vi "Calculate_Sensitivity.vi"(8 "Min Sensitivity":dbl, 9 "Current RPM":dbl, 10 "Max Sensitivity":dbl, 11 "Max RPM":dbl) -> (3 "Sensitivity":dbl)   [LabVIEW 2017]
panel:
  in  "stop":bool=TRUE
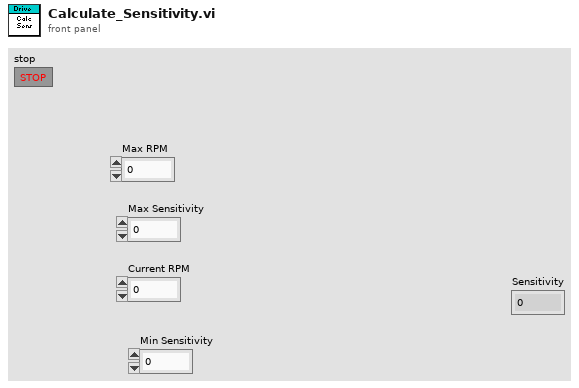
[diagram p1: front panel]
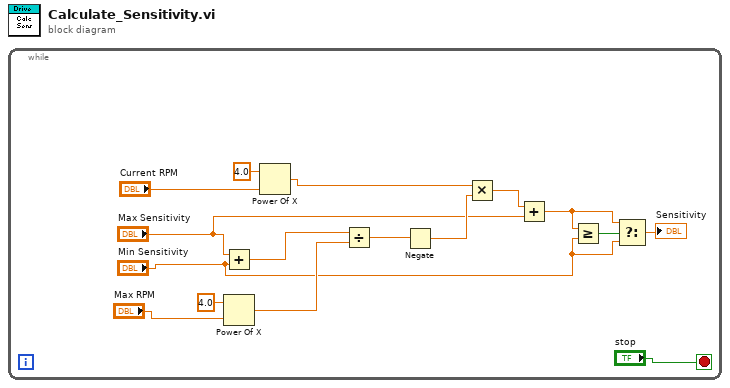
[diagram p0: block diagram]
diagram:
  n1 = while {
    stop <- "stop" stop-if-true
    n2 = Add(x="Max Sensitivity", y="Min Sensitivity") -> (x+y=w2:dbl)
    n3 = Power Of X(1:"Max RPM", 2:4.0 ("y")) -> (0:w15:dbl)
    n4 = Power Of X(1:"Current RPM", 2:4.0 ("y")) -> (0:w11:dbl)
    n5 = Divide(x=w2, y=w15) -> (x/y=w14:dbl)
    n6 = Negate(x=w14) -> (-x=w10:dbl)
    n7 = Multiply(x=w11, y=w10) -> (x*y=w9:dbl)
    n8 = Add(x=w9, y="Max Sensitivity") -> (x+y=w3:dbl)
    n9 = Greater Or Equal?(x=w3, y="Min Sensitivity") -> (x >= y?=w4:bool)
    n10 = Select(t=w3, s=w4, f="Min Sensitivity") -> (s? t:f=→"Sensitivity":dbl)
  }
